vi "VISA Connection Close.vi"(6 "Error In":errorcluster, 9 "VISA resource name":refnum<visa-resource-name>) -> (0 "Error Out":errorcluster)   [LabVIEW 2014, in "VISA Connection Template.lvlib"]
uses:
  VISA Connection Template.lvlib
panel:
  in  "Markers":T1
  out "RetData":string
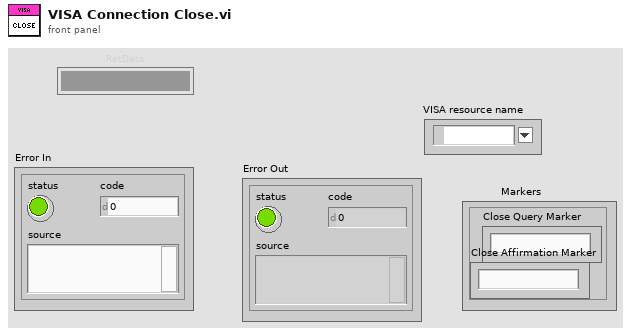
[diagram p1: front panel]
types:
  T1 = cluster{"Close Query Marker":string, "Close Affirmation Marker":string}
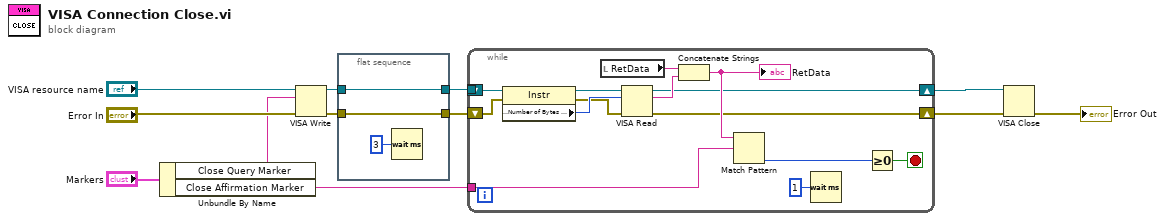
[diagram p0: block diagram]
diagram:
  n1 = Unbundle By Name("Markers") -> ("Close Query Marker"=w2:string, "Close Affirmation Marker"=w1:string)
  n2 = VISA Write(VISA resource name="VISA resource name", write buffer=w2, error in (no error)="Error In") -> (VISA resource name out=w11:refnum<visa-resource-name>, error out=w12:errorcluster)  [unwired: 1 out]
  n3 = flat-sequence {
    tunnel: w11 -> [w13]
    tunnel: [w14] -> w10
    tunnel: w12 -> [w14]
    tunnel: [w13] -> w4
    frame #0 {
      n4 = Wait (ms)(milliseconds to wait=u32 3) -> ()  [unwired: 1 out]
    }
  }
  n5 = while {
    shift-right: [w20] -> w6
    shift-left: _ -> [w21]
    shift-right: [w18] -> w7
    shift-left: w10 -> [w19]
    tunnel: w4 -> [_]
    tunnel: w1 -> [w16]
    stop <- w17 stop-if-true
    n6 = property class="Instr"(reference=w21, error in=w19) -> (reference out=w25:refnum<visa-resource-name>, error out=w22:errorcluster, "Serial Settings:Number of Bytes at Serial Port"=w24:u32)
    n7 = local read "RetData"() -> (w28:string)
    n8 = VISA Read(VISA resource name=w25, byte count=w24, error in (no error)=w22) -> (VISA resource name out=w20:refnum<visa-resource-name>, read buffer=w27:string, error out=w18:errorcluster)  [unwired: 1 out]
    n9 = Concatenate Strings(w28, w27) -> (w23:string)
    "RetData" <- w23
    n10 = Match Pattern(string=w23, regular expression=w16) -> (offset past match=w29:i32)  [unwired: 1 in, 3 out]
    n11 = Wait (ms)(milliseconds to wait=u32 1) -> ()  [unwired: 1 out]
    n12 = Greater Or Equal To 0?(x=w29) -> (x >= 0?=w17:bool)
  }
  n13 = VISA Close(VISA resource name=w6, error in (no error)=w7) -> (error out=→"Error Out":errorcluster)
